vi "Autonomous Test.vi"() -> ()   [LabVIEW 2013]
uses:
  Vision Data.vi
  <vilib>/Rock Robotics/WPI/RobotDrive/WPI_RobotDriveGetSetRefNum.vi
panel:
  in  "Hot Goal":bool
  out "Enum":T1(ring)
  out "Shot":bool
  in  "Desired Distance (in)":dbl
  in  "Deesired Distanc":i32(slide) scale=0.0..500.0
  out "Difference":i32(slide) scale=0.0..10.0
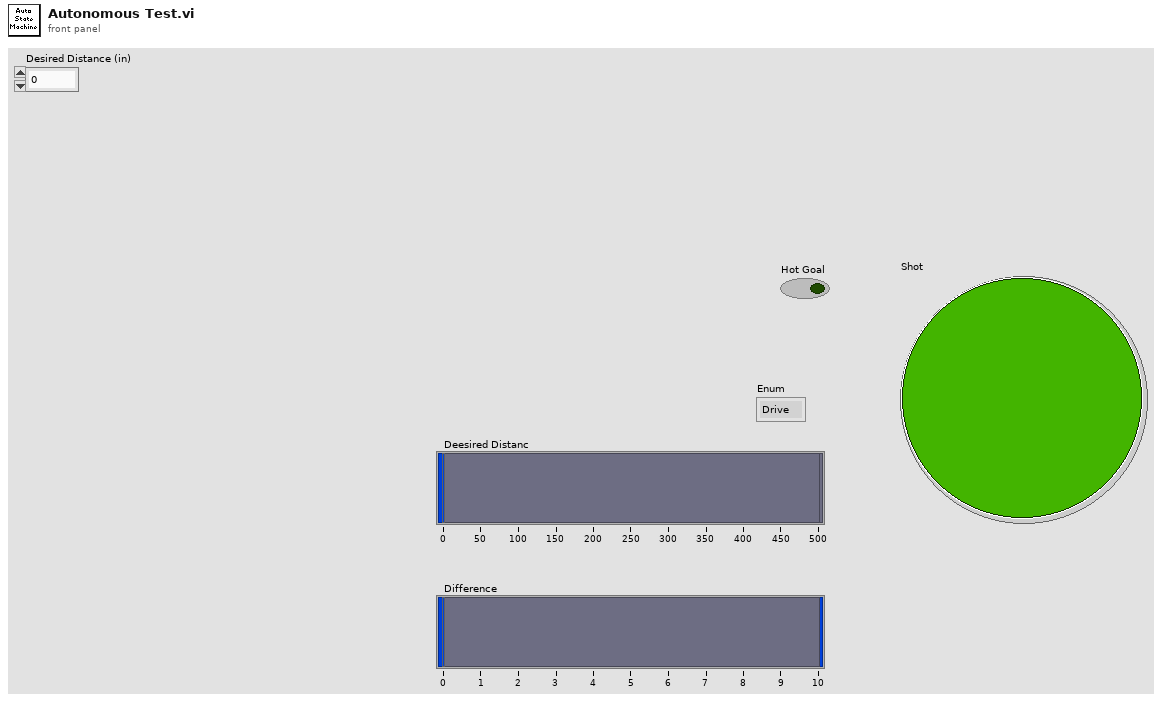
[diagram p1: front panel]
types:
  T1 = enum16{"Drive", "Wait", "Hot Goal Detection", "Shoot", "Turn Left", "Turn Right", "Turn 180"}
  T2 = typedef "WPI_RobotDriveDevRef.ctl" = cluster{"DevStatus":errorcluster, "Motors[]":T3[], "Square Inputs":bool, "Max Output":dbl, "Isochronous":bool}
  T3 = typedef "WPI_MotorControlDeviceRef.ctl" = cluster{"DeviceStatus":errorcluster, "Type":enum16{"PWM", "CAN"}, "PWM":cluster{"Digital Module":T4, "PWM Channel":T5, "DeadBand":T6}, "CAN":cluster{"Device Number":u8, "Control Mode":T7, "Semaphore":T8, "Max Vout":dbl}, "Invert":bool, "TransformRef":T9, "InvTransformRef":T9}
  T4 = typedef "FPGA_TypedefDigitalModule.ctl" = enum16{"Digital Module 1", "Digital Module 2"}
  T5 = typedef "FPGA_DIOPWMChannel.ctl" = enum8{"PWM 1", "PWM 2", "PWM 3", "PWM 4", "PWM 5", "PWM 6", "PWM 7", "PWM 8", "PWM 9", "PWM 10", "Invalid"}
  T6 = typedef "WPI_PWMDeadband.ctl" = cluster{"Name":string, "maxPositivePwm":i32, "minPositivePwm":i32, "centerPwm":i32, "maxNegativePwm":i32, "minNegativePwm":i32, "angularRange":u16}
  T7 = typedef "WPI_CANJaguar_ControlMode.ctl" = enum8{"Percent VBus", "Current", "Speed", "Position", "Voltage"}
  T8 = typedef "Semaphore RefNum" = refnum<k1>
  T9 = typedef "WPI_PWMTransform_ConPane.ctl" = refnum<vi>
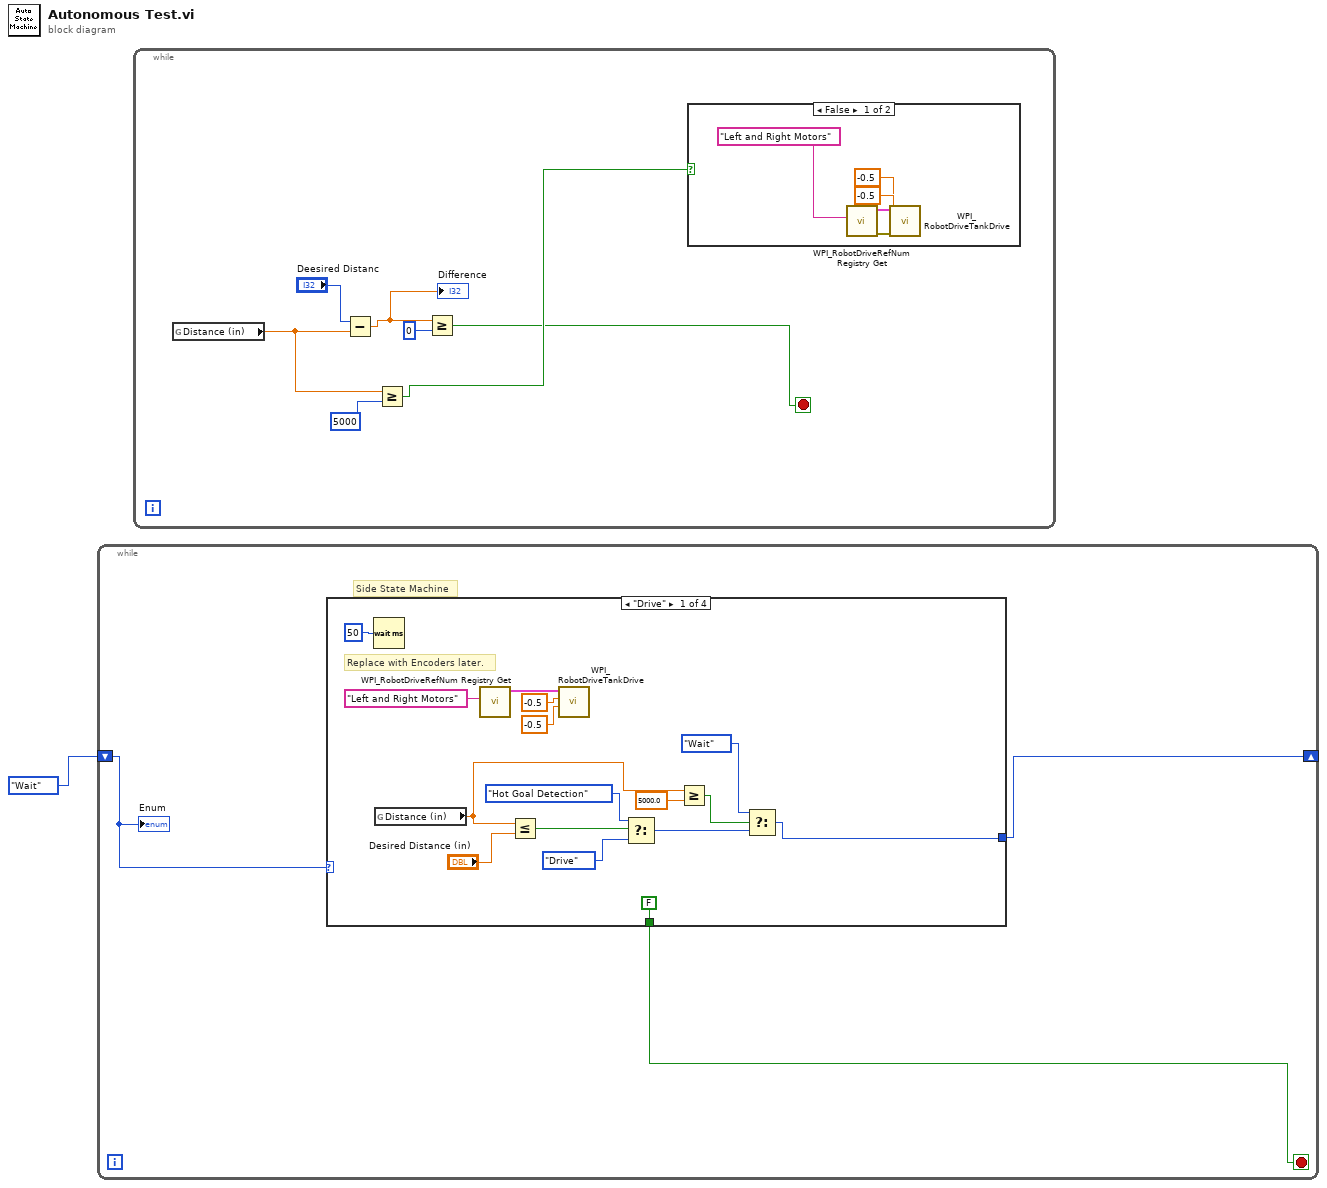
[diagram p0: block diagram]
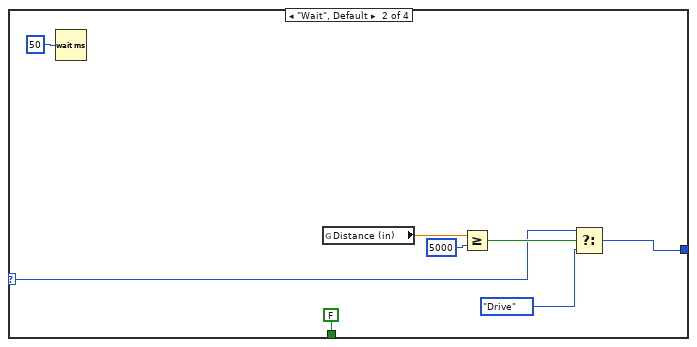
[diagram p2: hidden frame]
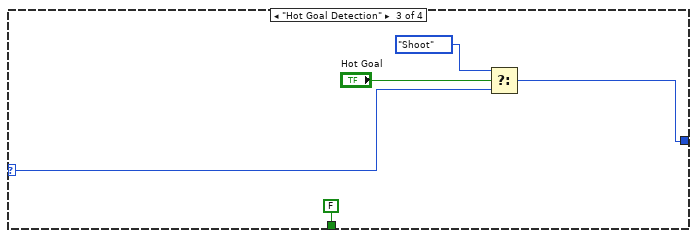
[diagram p3: hidden frame]
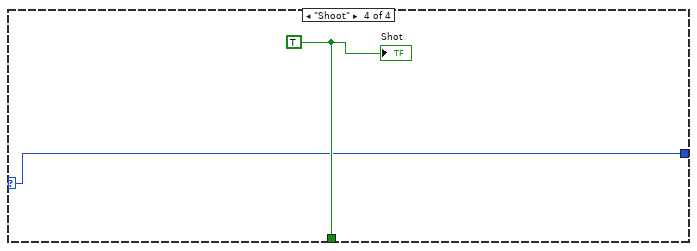
[diagram p4: hidden frame]
diagram:
  n1 = while {
    shift-right: [w3] -> _
    shift-left: T1."Wait" -> [w4]
    stop <- w2 stop-if-true
    # "Side State Machine"
    n2 = case shown="\"Drive\"" w4 {
      selector: w4 -> [_ w24 w32 w34]
      tunnel: [w6 w23 w31 w34] -> w3
      tunnel: [FALSE ("Shot") FALSE ("Shot") FALSE ("Shot") w35] -> w2
      frame "Drive" {
        # "Replace with Encoders later."
        n3 = Wait (ms)(milliseconds to wait=u32 50) -> ()  [unwired: 1 out]
        n4 = global read "Vision Data.vi" "Distance (in)"() -> (w10:dbl)
        n5 = call <vilib>:"WPI_RobotDriveRefNum Registry Get.vi"("refnum name"="Left and Right Motors") -> ("RobotDriveDevRef"=w16:T2)  [unwired: 9 in, 1 out]
        n6 = Less Or Equal?(x=w10, y="Desired Distance (in)") -> (x <= y?=w14:bool)
        n7 = call <vilib>:"WPI_RobotDriveTankDrive.vi"("Right axis value"=-0.5, "Left axis value"=-0.5, "RobotDriveDevRef"=w16) -> ()  [unwired: 6 in, 3 out]
        n8 = Select(t=T1."Hot Goal Detection", s=w14, f=T1."Drive") -> (s? t:f=w11:T1)
        n9 = Greater Or Equal?(x=w10, y=5000.0) -> (x >= y?=w8:bool)
        n10 = Select(t=T1."Wait", s=w8, f=w11) -> (s? t:f=w6:T1)
      }
      frame "Wait", Default {
        n11 = Wait (ms)(milliseconds to wait=u32 50) -> ()  [unwired: 1 out]
        n12 = global read "Vision Data.vi" "Distance (in)"() -> (w26:dbl)
        n13 = Greater Or Equal?(x=w26, y=5000) -> (x >= y?=w25:bool)
        n14 = Select(t=w24, s=w25, f=T1."Drive") -> (s? t:f=w23:T1)
      }
      frame "Hot Goal Detection" {
        n15 = Select(t=T1."Shoot", s="Hot Goal", f=w32) -> (s? t:f=w31:T1)
      }
      frame "Shoot" {
        w35 = TRUE ("Shot")
        "Shot" <- w35
      }
    }
    "Enum" <- w4
  }
  n16 = while {
    stop <- w36 stop-if-true
    n17 = global read "Vision Data.vi" "Distance (in)"() -> (w39:dbl)
    n18 = Subtract(x="Deesired Distanc", y=w39) -> (x-y=w40:dbl)
    "Difference" <- w40
    n19 = Greater Or Equal?(x=w39, y=5000) -> (x >= y?=w37:bool)
    n20 = Greater Or Equal?(x=w40, y=0) -> (x >= y?=w36:bool)
    n21 = case shown="False" w37 {
      frame False {
        n22 = call <vilib>:"WPI_RobotDriveRefNum Registry Get.vi"("refnum name"="Left and Right Motors") -> ("error out"=w47:errorcluster, "RobotDriveDevRef"=w46:T2)  [unwired: 9 in]
        n23 = call <vilib>:"WPI_RobotDriveTankDrive.vi"("error in (no error)"=w47, "Right axis value"=-0.5, "Left axis value"=-0.5, "RobotDriveDevRef"=w46) -> ()  [unwired: 5 in, 3 out]
      }
      frame True {
      }
    }
  }
